vi "S1500_S7Com_RW_1500.vi"(5 "Variant":variant, 8 "Fehler (Eingang)":errorcluster, 10 "connection ID IN":refnum<k5>, 11 "Variablen IN":T2={"DB"=0, "Adresse"=0, "Länge"=0, "Typ"=enum."BYTE", "Enum"=enum."WRITE"}) -> (0 "Fehler (Ausgang)":errorcluster, 2 "connection ID out":refnum<k5>, 3 "Read_Data":T1)   [LabVIEW 2018]
uses:
  S1500_ENUM Typ.ctl
  S1500_S7Com_DATATypes.ctl
  S1500_S7Com_RW.ctl
  S7Com_Source_inkl_IP/S7Com_Data_Array.ctl
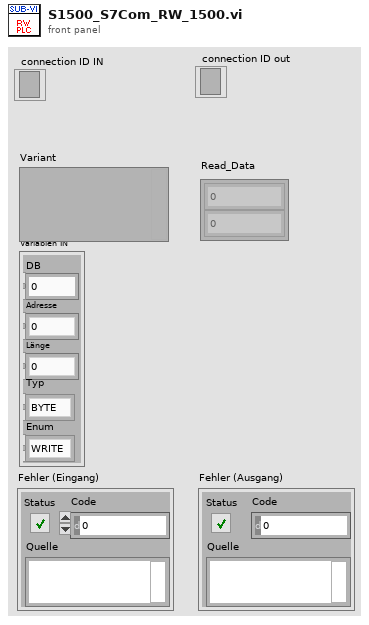
[diagram p1: front panel]
types:
  T1 = typedef "S7Com_Data_Array.ctl" = i32[]
  T2 = typedef "S1500_ENUM Typ.ctl" = cluster{"DB":u32, "Adresse":u32, "Länge":u32, "Typ":T3, "Enum":T4}
  T3 = typedef "S1500_S7Com_DATATypes.ctl" = enum16{"", "BIT", "BYTE", "CHAR", "WORD", "INT", "DWORD", "DINT", "REAL", "STRING"}
  T4 = typedef "S1500_S7Com_RW.ctl" = enum16{"WRITE", "READ"}
  T5 = typedef "S1500_S7Com_RW_CMD.ctl" = cluster{"Read Length":u16, "Data Block #":u16, "S7_Add_Area":T6, "Start Address":T7, "S7_Transport_Size":T8, "S7_Function":T9, "IP-Address":string}
  T6 = typedef "S1500_S7Com_Address_Area.ctl" = u8
  T7 = typedef "S1500_S7Com_Start_Add.ctl" = u16
  T8 = typedef "S1500_S7Com_Transport_Size.ctl" = u8
  T9 = typedef "S1500_S7Com_Function.ctl" = u8
  T10 = typedef "S1500_S7Com_Data_Array.ctl" = i32[]
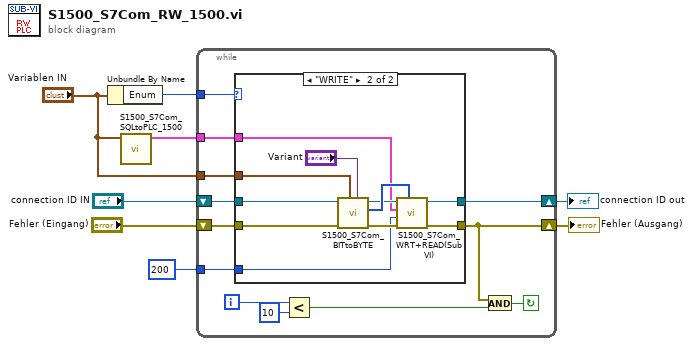
[diagram p0: block diagram]
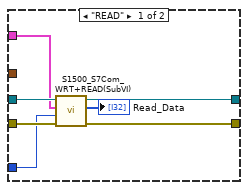
[diagram p2: hidden frame]
diagram:
  n1 = Unbundle By Name("Variablen IN") -> ("Enum"=w3:T4)
  n2 = call "S1500_S7Com_SQLtoPLC_1500.vi"("Variablen IN"="Variablen IN") -> ("RW_CMD"=w1:T5)  [unwired: 10 in]
  n3 = while {
    tunnel: 200 ("timeout ms (25000)") -> [w18]
    tunnel: w1 -> [w17]
    tunnel: "Variablen IN" -> [w16]
    tunnel: w3 -> [w15]
    shift-right: [w13] -> w4
    shift-left: "Fehler (Eingang)" -> [w19]
    shift-right: [w14] -> w7
    shift-left: "connection ID IN" -> [w20]
    i -> [w10]
    stop <- w12 continue-if-true
    n4 = case shown="\"WRITE\"" w15 {
      tunnel: w19 -> [w27 w30]
      tunnel: w20 -> [w26 w29]
      tunnel: w17 -> [w21 w28]
      tunnel: [w25 w37] -> w13
      tunnel: w18 -> [w24 w32]
      tunnel: w16 -> [_ w33]
      tunnel: [w23 w31] -> w14
      frame "READ" {
        n5 = call "S1500_S7Com_WRT+READ(SubVI).vi"("error in"=w27, "timeout ms (25000)"=w24, "RW_CMD"=w21, "connection ID in"=w26) -> ("error out"=w25:errorcluster, "Read_Data"=→"Read_Data":T10, "connection ID out"=w23:refnum<k5>)  [unwired: 1 in, 1 out]
      }
      frame "WRITE" {
        n6 = call "S1500_S7Com_BITtoBYTE.vi"("Variant"="Variant", "Cluster"=w33, "error in"=w30) -> ("error out"=w36:errorcluster, "RW Data"=w35:i32[])  [unwired: 7 in]
        n7 = call "S1500_S7Com_WRT+READ(SubVI).vi"("Write_Data"=w35, "error in"=w36, "timeout ms (25000)"=w32, "RW_CMD"=w28, "connection ID in"=w29) -> ("error out"=w37:errorcluster, "connection ID out"=w31:refnum<k5>)  [unwired: 2 out]
      }
    }
    n8 = Less?(x=w10, y=10 ("x")) -> (x < y?=w9:bool)
    n9 = And(x=w13, y=w9) -> (x .and. y?=w12:bool)
  }
  "Fehler (Ausgang)" <- w4
  "connection ID out" <- w7
